vi "Strip apostrophe.vi"   [LabVIEW 2017, in "_lvcicd_support_2017.lvlib"]
uses:
  _lvcicd_support_2017.lvlib
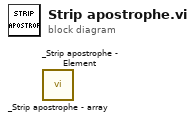
[diagram p0: block diagram]
diagram:
  n1 = call "_Strip apostrophe - array.vi"() -> ()  [unwired: 11 in, 1 out]
  n2 = call "_Strip apostrophe - Element.vi"() -> ()  [unwired: 11 in, 1 out]
